vi "_HexStrPtr To FlattenStrPtr.vi"(1 "HexStrPtr":string) -> (0 "FlattenStrPtr":string)   [LabVIEW 2014]
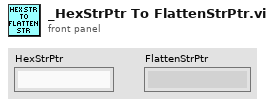
[diagram p1: front panel]
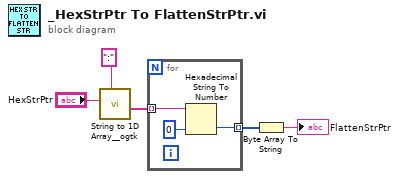
[diagram p0: block diagram]
diagram:
  n1 = call <userlib>:"String to 1D Array__ogtk.vi"("delimiter (Tab)"=":", "string"="HexStrPtr") -> ("Array of Strings"=w3:string[])  [unwired: 9 in]
  n2 = for {
    tunnel: w3 -> [w8] mode=indexing
    tunnel: [w7] -> w5 mode=indexing
    n3 = Hexadecimal String To Number(string=w8, default (0uL)=u8 0 ("default (0 U32)")) -> (number=w7:u8)  [unwired: 1 in, 1 out]
  }
  n4 = Byte Array To String(unsigned byte array=w5) -> (string=→"FlattenStrPtr":string)
